vi "uc480_SubVI_Example_Trigger.vi"(0 ".NET (Reference)":refnum<k24>, 5 "Trigger Mode":u8, 7 "Trigger Delay":i32, 9 "Trigger Debounce":i32, 11 "Error In":errorcluster) -> (4 "Trigger Mode":i32, 15 "Error Out":errorcluster)   [LabVIEW 2011]
uses:
  C:/Program Files/Thorlabs/Scientific Imaging/DCx Camera Support/Develop/DotNet/uc480DotNet.dll
  Develop/DotNet/uc480DotNet.dll
  C:/Program Files/IDS/uEye/OtherDrivers/LabVIEW/ueye.NET/uEyeDotNet.dll
  IDS/uEye/OtherDrivers/LabVIEW/ueye.NET/uEyeDotNet.dll
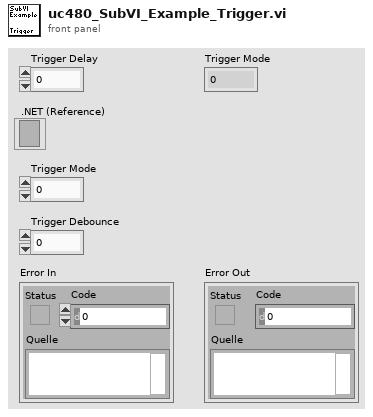
[diagram p1: front panel]
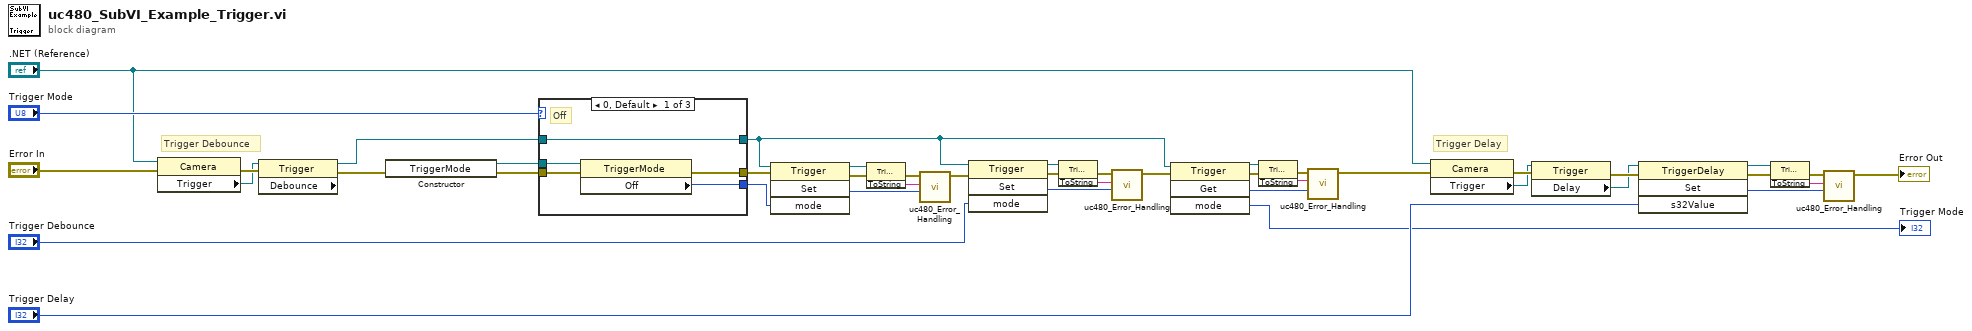
[diagram p0: block diagram]
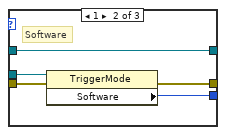
[diagram p2: hidden frame]
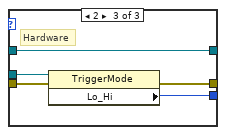
[diagram p3: hidden frame]
diagram:
  # "Trigger Debounce"
  # "Trigger Delay"
  n1 = property on="Eigenschaftsknoten" class="Camera"(reference=".NET (Reference)", error in="Error In") -> (error out=w13:errorcluster, "Trigger"=w12:refnum<k24>)  [unwired: 1 out]
  n2 = property class="Trigger" props=["Debounce"](reference=w12, error in=w13) -> (reference out=w15:refnum<k24>, error out=w14:errorcluster)  [unwired: 1 out]
  n3 = constructor class="TriggerMode"(error in=w14) -> (reference out=w5:refnum<k24>, error out=w6:errorcluster)  [unwired: 2 in, 1 out]
  n4 = case shown="0, Default" "Trigger Mode" {
    tunnel: w5 -> [w48 w52 w57]
    tunnel: w6 -> [w47 w51 w56]
    tunnel: w15 -> [w46 w53 w58]
    tunnel: [w46 w53 w58] -> w3
    tunnel: [w45 w49 w55] -> w16
    tunnel: [w44 w50 w54] -> w22
    frame 0, Default {
      # "Off"
      n5 = property class="TriggerMode"(reference=w48, error in=w47) -> (error out=w45:errorcluster, "Off"=w44:i32)  [unwired: 1 out]
    }
    frame 1 {
      # "Software"
      n6 = property class="TriggerMode"(reference=w52, error in=w51) -> (error out=w49:errorcluster, "Software"=w50:i32)  [unwired: 1 out]
    }
    frame 2 {
      # "Hardware"
      n7 = property class="TriggerMode"(reference=w57, error in=w56) -> (error out=w55:errorcluster, "Lo_Hi"=w54:i32)  [unwired: 1 out]
    }
  }
  n8 = invoke class="Trigger" method="Set"(reference=w3, error in=w16, "mode"=w22) -> (reference out=w9:refnum<k24>, error out=w8:errorcluster, "Set"=w7:i32)  [unwired: 1 in, 1 out]
  n9 = invoke class="Trigger" method="ToString"(reference=w9, error in=w8) -> (error out=w11:errorcluster, "ToString"=w10:string)  [unwired: 1 in, 1 out]
  n10 = call "uc480_Error_Handling.vi"("Error Code"=w7, "Error String"=w10, "Error In"=w11) -> ("Error Out"=w39:errorcluster)  [unwired: 8 in]
  n11 = invoke class="Trigger" method="Set"(reference=w3, error in=w39, "mode"="Trigger Debounce") -> (reference out=w36:refnum<k24>, error out=w37:errorcluster, "Set"=w38:i32)  [unwired: 1 in, 1 out]
  n12 = invoke class="Trigger" method="ToString"(reference=w36, error in=w37) -> (error out=w35:errorcluster, "ToString"=w34:string)  [unwired: 1 in, 1 out]
  n13 = call "uc480_Error_Handling.vi"("Error Code"=w38, "Error String"=w34, "Error In"=w35) -> ("Error Out"=w40:errorcluster)  [unwired: 8 in]
  n14 = invoke class="Trigger" method="Get"(reference=w3, error in=w40) -> (reference out=w28:refnum<k24>, error out=w29:errorcluster, "Get"=w30:i32, "mode"=→"Trigger Mode":i32)  [unwired: 2 in]
  n15 = invoke class="Trigger" method="ToString"(reference=w28, error in=w29) -> (error out=w32:errorcluster, "ToString"=w31:string)  [unwired: 1 in, 1 out]
  n16 = call "uc480_Error_Handling.vi"("Error Code"=w30, "Error String"=w31, "Error In"=w32) -> ("Error Out"=w43:errorcluster)  [unwired: 8 in]
  n17 = property on="Eigenschaftsknoten" class="Camera"(reference=".NET (Reference)", error in=w43) -> (error out=w18:errorcluster, "Trigger"=w2:refnum<k24>)  [unwired: 1 out]
  n18 = property class="Trigger"(reference=w2, error in=w18) -> (error out=w20:errorcluster, "Delay"=w19:refnum<k24>)  [unwired: 1 out]
  n19 = invoke class="TriggerDelay" method="Set"(reference=w19, error in=w20, "s32Value"="Trigger Delay") -> (reference out=w25:refnum<k24>, error out=w26:errorcluster, "Set"=w27:i32)  [unwired: 1 in, 1 out]
  n20 = invoke class="TriggerDelay" method="ToString"(reference=w25, error in=w26) -> (error out=w24:errorcluster, "ToString"=w23:string)  [unwired: 1 in, 1 out]
  n21 = call "uc480_Error_Handling.vi"("Error Code"=w27, "Error String"=w23, "Error In"=w24) -> ("Error Out"=→"Error Out":errorcluster)  [unwired: 8 in]
